vi "Verify Display.vi"(0 "GEA2 Reference In":refnum<k24>, 5 "Expected LEDs":T1, 7 "Care?":T8, 9 "Ignore Brightness?":bool, 11 "Error In":errorcluster) -> (4 "GEA2 Reference Out":refnum<k24>, 6 "Pass/Fail?":bool, 8 "Report Text":string, 15 "Error Out":errorcluster)   [LabVIEW 2016, in "TLMB.lvlib"]
doc: "This VI is used to verify the display on the HEUI."
uses:
  Projects/TLMB.lvlib
  Q:/Common/DLLs/GEA3/GeaCommunication.dll
  Common/DLLs/GEA3/GeaCommunication.dll
  controls/HEUI_Display_Care.ctl
  controls/HEUI_Display.ctl
  controls/Cycle Selection Enum.ctl
  controls/Stain Enum.ctl
  controls/Temp Enum.ctl
  controls/Soil Enum.ctl
  controls/Spin Enum.ctl
  controls/750 Status Enum.ctl
  Common/LabVIEW GEA2 Toolkit/LabVIEW_GEA2_Toolkit.lvlibp/type defs/Source_Destination.ctl
  Common/LabVIEW GEA2 Toolkit/LabVIEW_GEA2_Toolkit.lvlibp/type defs/ERD Read Data In.ctl
  Common/LabVIEW GEA2 Toolkit/LabVIEW_GEA2_Toolkit.lvlibp/type defs/Data Type.ctl
  Common/LabVIEW GEA2 Toolkit/LabVIEW_GEA2_Toolkit.lvlibp
panel:
  in  "Standalone?":bool
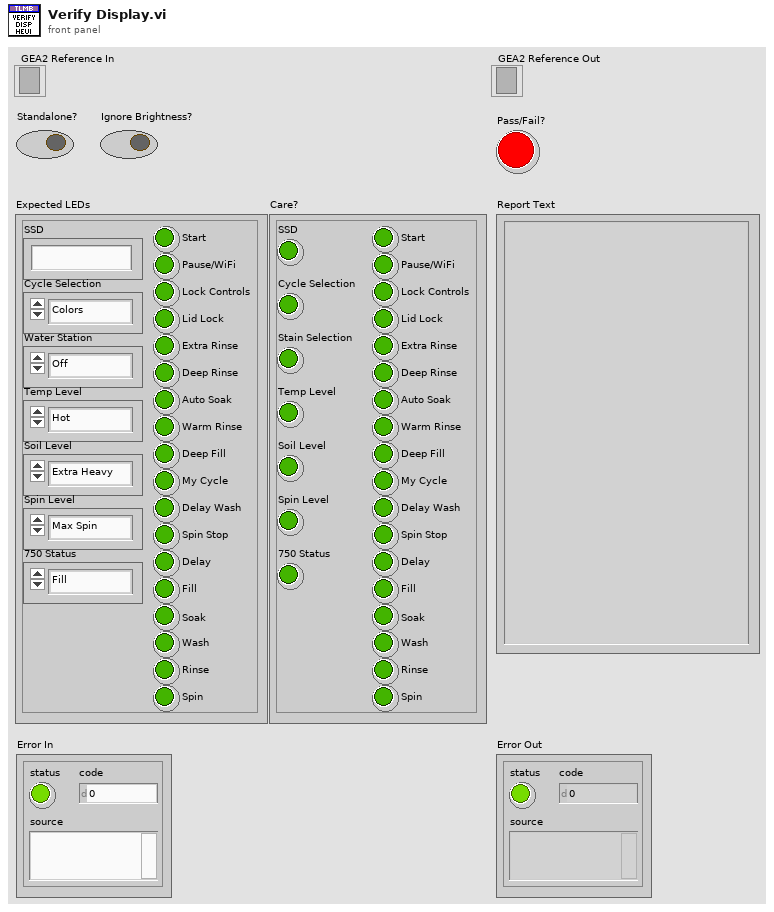
[diagram p1: front panel]
types:
  T1 = typedef "TLMB.lvlib/HEUI_Display.ctl" = cluster{"SSD":string, "Cycle Selection":T2, "Water Station":T3, "Temp Level":T4, "Soil Level":T5, "Spin Level":T6, "750 Status":T7, "Start":bool, "Pause/WiFi":bool, "Lock Controls":bool, "Lid Lock":bool, "Extra Rinse":bool, "Deep Rinse":bool, "Auto Soak":bool, "Warm Rinse":bool, "Deep Fill":bool, "My Cycle":bool, "Delay Wash":bool, "Spin Stop":bool, "Delay":bool, "Fill":bool, "Soak":bool, "Wash":bool, "Rinse":bool, "Spin":bool}
  T2 = typedef "TLMB.lvlib/Cycle Selection Enum.ctl" = enum16{"Colors", "Easy Care", "Delicates", "Hand Wash", "Active Wear", "Speed Wash", "Rinse and Spin", "Drain and Spin", "Basket Clean", "Jeans", "Heavy Duty", "Bulky Items", "Towels", "Whites", "Off", "*Incorrect*"}
  T3 = typedef "TLMB.lvlib/Stain Enum.ctl" = enum16{"Off", "Water", "Water & Detergent", "*Incorrect*"}
  T4 = typedef "TLMB.lvlib/Temp Enum.ctl" = enum16{"Hot", "Warm", "Colors", "Cool", "Cold", "Tap Cold", "Off", "*Incorrect*"}
  T5 = typedef "TLMB.lvlib/Soil Enum.ctl" = enum16{"Extra Heavy", "Heavy", "Normal", "Light", "Off", "*Incorrect*"}
  T6 = typedef "TLMB.lvlib/Spin Enum.ctl" = enum16{"Max Spin", "More Spin", "Normal Spin", "No Spin", "Off", "*Incorrect*"}
  T7 = typedef "TLMB.lvlib/750 Status Enum.ctl" = enum16{"Fill", "Wash", "Rinse", "Spin", "Off", "*Incorrect*"}
  T8 = typedef "TLMB.lvlib/HEUI_Display_Care.ctl" = cluster{"SSD":bool, "Cycle Selection":bool, "Stain Selection":bool, "Temp Level":bool, "Soil Level":bool, "Spin Level":bool, "750 Status":bool, "Start":bool, "Pause/WiFi":bool, "Lock Controls":bool, "Lid Lock":bool, "Extra Rinse":bool, "Deep Rinse":bool, "Auto Soak":bool, "Warm Rinse":bool, "Deep Fill":bool, "My Cycle":bool, "Delay Wash":bool, "Spin Stop":bool, "Delay":bool, "Fill":bool, "Soak":bool, "Wash":bool, "Rinse":bool, "Spin":bool}
  T9 = typedef "LabVIEW_GEA2_Toolkit.lvlibp/ERD Read Data In.ctl" = cluster{"ERD Number":u16, "Data Type":T10}
  T10 = typedef "LabVIEW_GEA2_Toolkit.lvlibp/Data Type.ctl" = enum16{"string", "boolean", "uint8_t", "uint16_t", "uint32_t", "uint64_t", "int8_t", "int16_t", "int32_t", "int64_t"}
  T11 = typedef "LabVIEW_GEA2_Toolkit.lvlibp/Source_Destination.ctl" = cluster{"Source":u8, "Destination":u8}
  T12 = typedef "TLMB.lvlib/HEUI_LEDs.ctl" = cluster{"Z101 - Start":bool, "Z103 - Colors":bool, "Z104 - Whites":bool, "Z105 - Towels":bool, "Z106 - Bulky Items":bool, "Z107 - Heavy Duty":bool, "Z108 - Jeans":bool, "Z109 - Basket Clean":bool, "Z110 - Drain and Spin":bool, "Z111 - Rinse and Spin":bool, "Z112 - Speed Wash":bool, "Z113 - Active Wear":bool, "Z114 - Hand Wash":bool, "Z115 - Delicates":bool, "Z116 - Easy Care":bool, "Z117 - Tomato":bool, "Z118 - Wine":bool, "Z119 - Blood":bool, "Z120 - Grass":bool, "Z121 - Dirt":bool, "Z122_MSB_A":bool, "Z123_MSB_B":bool, "Z124_MSB_G":bool, "Z125_MSB_C":bool, "Z126_MSB_D":bool, "Z127_MSB_E":bool, "Z128_MSB_F":bool, "Z129_LSB_A":bool, "Z130_LSB_B":bool, "Z131_LSB_G":bool, "Z132_LSB_C":bool, "Z133_LSB_D":bool, "Z134_LSB_E":bool, "Z135_LSB_F":bool, "Z136 - Pause":bool, "Z137 - Pause":bool, "Z138 - Lock Controls":bool, "Z139 - Lock Controls":bool, "Z140 - Lock Controls":bool, "Z141 - Lid Lock":bool, "Z142 - Lid Lock":bool, "Z143 - Lid Lock":bool, "Z144 - Good":bool, "Z145":bool, "Z146":bool, "Z147 - Better":bool, "Z148 - Delay":bool, "Z149 - Fill":bool, "Z150 - Soak":bool, "Z151 - Wash":bool, "Z152 - Rinse":bool, "Z153 - Spin":bool, "Z154 - Hot":bool, "Z155 - Warm":bool, "Z156 - Colors":bool, "Z157 - Cool":bool, "Z158 - Cold":bool, "Z159 - Tap Cold":bool, "Z160 - Extra Heavy":bool, "Z161 - Heavy":bool, "Z162 - Normal":bool, "Z163 - Light":bool, "Z164 - Max Spin":bool, "Z165 - More Spin":bool, "Z166 - Normal Spin":bool, "Z167 - No Spin":bool, "Z168 - Extra Rinse":bool, "Z170 - Deep Rinse":bool, "Z171 - Auto Soak":bool, "Z172 - Warm Rinse":bool, "Z173 - Deep Fill":bool, "Z174 - My Cycles":bool, "Z175 - Delay Wash":bool, "Z176 - Spin Stop":bool, "Z177 - Spin Stop":bool, "Z178 - Spin Stop":bool, "Z179 - Pause":bool, "Z109":bool, "Z110":bool, "Z123":bool, "Z124":bool, "Z140":bool, "Unused0":bool, "Unused1":bool, "Unused2":bool, "Unused3":bool, "Channel_Off":bool, "Channel_Cycle_Unmapped":bool}
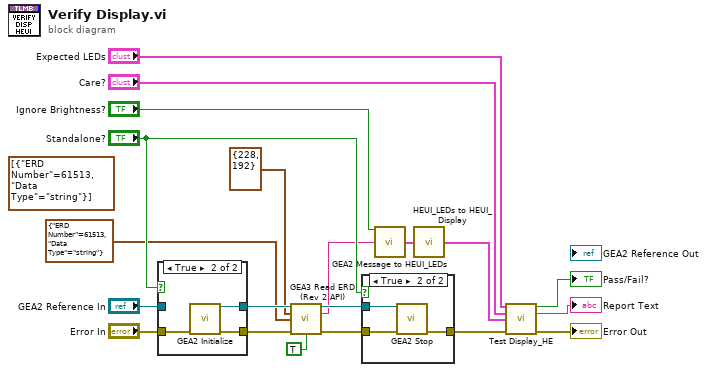
[diagram p0: block diagram]
diagram:
  (unwired) T9[] [{"ERD Number"=61513, "Data Type"=enum."string"}] ("Read ERD List")
  n1 = case shown="True" "Standalone?" {
    tunnel: [w21 w25] -> w4
    tunnel: "Error In" -> [w21 w24]
    tunnel: [w22 w23] -> w8
    tunnel: "GEA2 Reference In" -> [w22 _]
    frame False {
    }
    frame True {
      n2 = call "GEA2 Initialize.vi"("error in"=w24) -> ("GEA2 Reference Out"=w23:refnum<k24>, "error out"=w25:errorcluster)  [unwired: 12 in, 1 out]
    }
  }
  n3 = call "GEA3 Read ERD (Rev 2 API).vi"("GEA2 Reference In"=w8, "GEA Inputs"=T11 {"Source"=228, "Destination"=192}, "ERD Read Data In"=T9 {"ERD Number"=61513, "Data Type"=enum."string"}, "Error In"=w4, "Verify ERD Response?"=TRUE) -> ("GEA2 Reference Out"=w7:refnum<k24>, "Raw Data Out"=w1:string, "Error Out"=w3:errorcluster)  [unwired: 7 in, 1 out]
  n4 = case shown="True" "Standalone?" {
    tunnel: [_ w28] -> w13
    tunnel: w7 -> [_ w27]
    tunnel: w3 -> [_ w26]
    frame False {
    }
    frame True {
      n5 = call "GEA2 Stop.vi"("GEA2 Reference In"=w27, "Error In"=w26) -> ("Error Out"=w28:errorcluster)  [unwired: 13 in]
    }
  }
  n6 = call "GEA2 Message to HEUI_LEDs.vi"("Ignore Brightness?"="Ignore Brightness?", "Raw Data In"=w1) -> ("HEUI_LEDs"=w11:T12)  [unwired: 13 in]
  n7 = call "HEUI_LEDs to HEUI_Display.vi"("HEUI_LEDs"=w11) -> ("HEUI_Display"=w10:T1)  [unwired: 14 in]
  n8 = call "Test Display_HE.vi"("Expected LEDs"="Expected LEDs", "Care?"="Care?", "Actual LEDs"=w10, "error in"=w13) -> ("Pass/Fail?"=→"Pass/Fail?":bool, "Report Text"=→"Report Text":string, "error out"=→"Error Out":errorcluster)  [unwired: 9 in]
